vi "Initialise.vi"(6 "Diffuse Colour":refnum<vi>, 8 "error in (no error)":errorcluster, 10 "Resource Directory":path, 11 "Screen Dimensions":T1={"Width"=800, "Height"=600}) -> (0 "error out":errorcluster, 3 "Scene out":refnum<class "Scene.lvclass">)   [LabVIEW 2020, in "Application.lvlib" / "Scene.lvclass"]
uses:
  Scene.lvclass
  Libraries/Raster/Rectangle Dimensions.ctl
  Libraries/3D/Camera.ctl
  Camera.ctl
  Scene.lvclass/Scene.ctl
  Libraries/3D/Calculate A F Q.vi
  Libraries/3D/Degrees To Radians.vi
  Libraries/3D/3D.lvlib
  Application.lvlib
  Libraries/Raster/Raster.lvlib
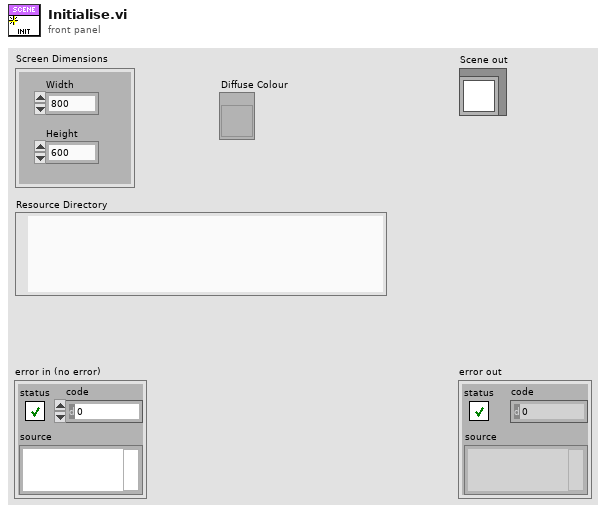
[diagram p1: front panel]
types:
  T1 = typedef "Raster.lvlib/Rectangle Dimensions.ctl" = cluster{"Width":u32, "Height":u32}
  T2 = typedef "Application.lvlib/Camera.ctl" = cluster{"Up":sgl, "Left":sgl, "Rotation":sgl, "Forward":sgl}
  T3 = typedef "3D.lvlib/Camera.ctl" = cluster{"Field Of View":sgl, "Near Plane":sgl, "Far Plane":sgl}
  T4 = typedef "3D.lvlib/Object.ctl" = cluster{"Triangles":T5[], "Transform":T11, "Name":string, "Alpha Blending Enabled":bool, "Alpha":dbl, "Turntable Enabled":bool, "Material":T9}
  T5 = typedef "3D.lvlib/Triangle.ctl" = cluster{"Vertex 1":T6, "Vertex 2":T6, "Vertex 3":T6, "Alpha":dbl, "Alpha Blending Enabled":bool, "Colour":u32, "Material":T9}
  T6 = typedef "3D.lvlib/Vertex.ctl" = cluster{"Position":T7, "UV":T8, "Colour":u32}
  T7 = typedef "3D.lvlib/Vector 3D.ctl" = cluster{"x":sgl, "y":sgl, "z":sgl}
  T8 = typedef "Raster.lvlib/UV.ctl" = cluster{"u":sgl, "v":sgl}
  T9 = typedef "3D.lvlib/Material.ctl" = cluster{"Diffuse Colour":u32, "Texture":T10}
  T10 = typedef "Raster.lvlib/Texture.ctl" = cluster{"Pixels":refnum<data-value>, "Size":T1}
  T11 = typedef "3D.lvlib/Transform.ctl" = cluster{"Position":T7, "Rotation":T7, "Scale":T7}
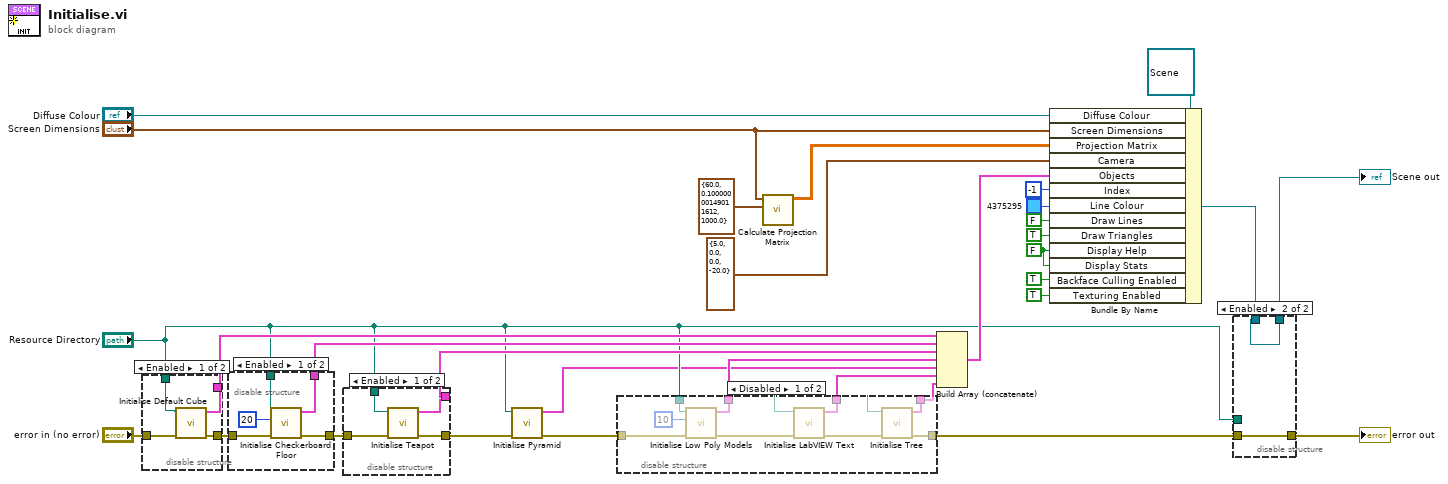
[diagram p0: block diagram]
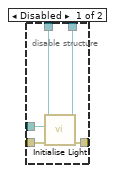
[diagram p3: hidden frame]
diagram:
  w7 = FALSE ("Display Help")
  n1 = disable-structure shown="Enabled" {
    disable-tunnel: "error in (no error)" -> [w35 _]
    disable-tunnel: [w34 _] -> w9
    disable-tunnel: [w33 _] -> w8
    disable-tunnel: "Resource Directory" -> [w32 _]
    frame Enabled {
      n2 = call "Initialise Default Cube.vi"("error in (no error)"=w35, "Resource Directory"=w32) -> ("error out"=w34:errorcluster, "Cube"=w33:T4)  [unwired: 8 in]
    }
    frame Disabled {
    }
  }
  n3 = disable-structure shown="Enabled" {
    disable-tunnel: [w40 _] -> w26
    disable-tunnel: [w38 w41] -> w24
    disable-tunnel: w9 -> [w37 w41]
    disable-tunnel: "Resource Directory" -> [w36 _]
    frame Enabled {
      n4 = call "Initialise Checkerboard Floor.vi"("error in (no error)"=w37, "Number Of Squares Per Side"=20, "Resource Directory"=w36) -> ("error out"=w38:errorcluster, "Checkerboard Floor"=w40:T4[])  [unwired: 7 in]
    }
    frame Disabled {
    }
  }
  n5 = disable-structure shown="Enabled" {
    disable-tunnel: w24 -> [w45 w46]
    disable-tunnel: [w44 w46] -> w5
    disable-tunnel: [w43 _] -> w23
    disable-tunnel: "Resource Directory" -> [w42 _]
    frame Enabled {
      n6 = call "Initialise Teapot.vi"("error in (no error)"=w45, "Resource Directory"=w42) -> ("error out"=w44:errorcluster, "Teapot"=w43:T4)  [unwired: 8 in]
    }
    frame Disabled {
    }
  }
  n7 = call "Initialise Pyramid.vi"("error in (no error)"=w5, "Resource Directory"="Resource Directory") -> ("error out"=w3:errorcluster, "Teapot"=w2:T4)  [unwired: 8 in]
  n8 = disable-structure shown="Disabled" {
    disable-tunnel: w3 -> [w54 w56]
    disable-tunnel: [w53 _] -> w22
    disable-tunnel: [w51 _] -> w16
    disable-tunnel: [w49 w56] -> w15
    disable-tunnel: [w48 _] -> w14
    disable-tunnel: "Resource Directory" -> [w47 _]
    frame Disabled {
      n9 = call "Initialise Low Poly Models.vi"("error in (no error)"=w54, "Number Of Objects"=10 ("Number Of Cubes"), "Resource Directory"=w47) -> ("error out"=w52:errorcluster, "Cubes"=w53:T4[])  [unwired: 7 in]
      n10 = call "Initialise LabVIEW Text.vi"("error in (no error)"=w52, "Resource Directory"=w47) -> ("error out"=w50:errorcluster, "Teapot"=w51:T4)  [unwired: 8 in]
      n11 = call "Initialise Tree.vi"("error in (no error)"=w50, "Resource Directory"=w47) -> ("error out"=w49:errorcluster, "Teapot"=w48:T4)  [unwired: 8 in]
    }
    frame Enabled {
    }
  }
  n12 = call "Calculate Projection Matrix.vi"("Camera"=T3 {"Field Of View"=60.0, "Near Plane"=0.1, "Far Plane"=1000.0}, "Screen Dimensions"="Screen Dimensions") -> ("Projection Matrix"=w28:sgl[][])  [unwired: 9 in]
  n13 = Build Array (concatenate)(w8, w26, w23, w22, w2, w16, w14) -> (w21:T4[])
  n14 = Bundle By Name(cluster=refnum<class "Scene.lvclass"> refnum ("Scene in"), "Diffuse Colour"="Diffuse Colour", "Screen Dimensions"="Screen Dimensions", "Projection Matrix"=w28, "Camera"=T2 {"Up"=5.0, "Left"=0.0, "Rotation"=0.0, "Forward"=-20.0}, "Objects"=w21, "Index"=-1 ("Active Object"), "Line Colour"=u32 4375295, "Draw Lines"=FALSE, "Draw Triangles"=TRUE, "Display Help"=w7, "Display Stats"=w7, "Backface Culling Enabled"=TRUE ("Display Help"), "Texturing Enabled"=TRUE) -> (w19:refnum<class "Scene.lvclass">)
  n15 = disable-structure shown="Enabled" {
    disable-tunnel: [w61 w62] -> w20
    disable-tunnel: w19 -> [w60 w63]
    disable-tunnel: [w59 w63] -> w18
    disable-tunnel: w15 -> [w58 w62]
    disable-tunnel: "Resource Directory" -> [w57 _]
    frame Disabled {
      n16 = call "Initialise Light.vi"("error in (no error)"=w58, "Resource Directory"=w57, "Scene in"=w60) -> ("error out"=w61:errorcluster, "Scene out"=w59:refnum<class "Scene.lvclass">)  [unwired: 7 in]
    }
    frame Enabled {
    }
  }
  "error out" <- w20
  "Scene out" <- w18
